vi "Do.vi"(8 "Error In":errorcluster, 10 "Actor in":refnum<class "Actor.lvclass">, 11 "CS++LNAMessage":refnum<class "CS++LNAMessage.lvclass">) -> (0 "Error Out":errorcluster, 2 "Actor out":refnum<class "Actor.lvclass">)   [LabVIEW 2016, in "CS++LNA.lvlib" / "CS++LNAMessage.lvclass"]
doc: "This VI creates the desired message object as class default object. Derives message classes need to override the <b>Parameter to Attribute.vi</b> to parse the variant attributes to the message object attribute.\n\nVI-Parameter Names of corresponding public VI of the derived actor class = Variant Attribute Names\n\nErrors (-8990, -8991, -8992) need to be handled in actor's <b>Handle Error.vi</b>\n\n(<B>Filename</B>: Actor Framework.lvlib:Message.lvclass:Do.vi)\n\nDefines what a message does when it is received by an actor. Generally, a message instructs an actor to invoke one of its methods. By default, this method does nothing. A child class must override it to define behavior. Create a child class by using the Actor Framework Message Maker dialog box."
uses:
  CS++LNAMessage.lvclass
  <vilib>/ActorFramework/Actor/Actor.lvclass
  <vilib>/ActorFramework/Message/Message.lvclass
  CS++LNAMessage.lvclass/CS++LNAMessage.ctl
  CS++LNAReturnMessage/CS++LNAReturnMessage.lvclass
  CSPP_Core/Libraries/Utilities/CS++Utilities.lvlib
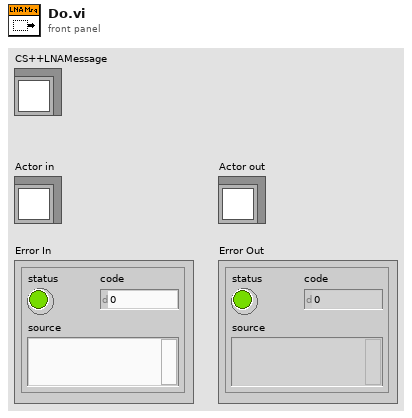
[diagram p1: front panel]
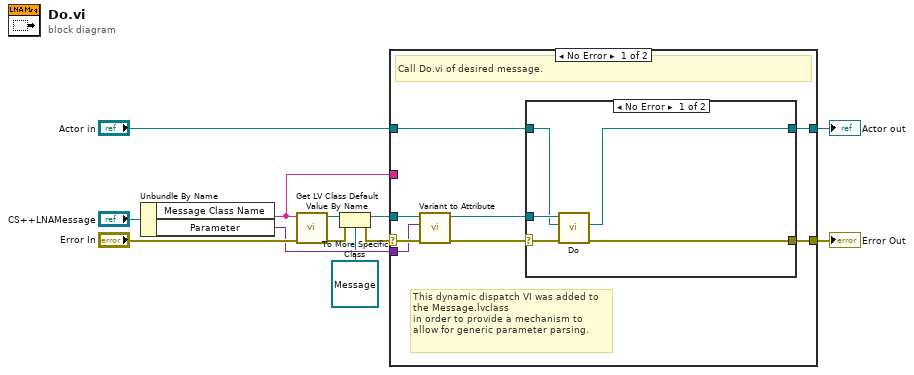
[diagram p0: block diagram]
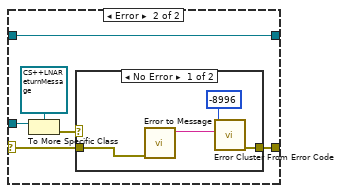
[diagram p2: hidden frame]
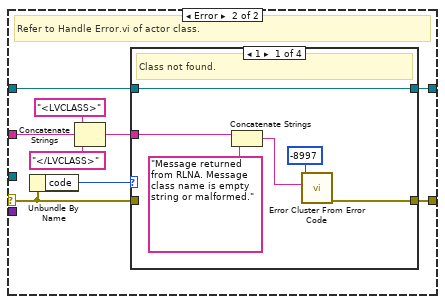
[diagram p4: hidden frame]
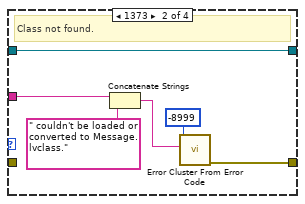
[diagram p5: hidden frame]
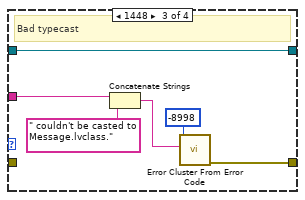
[diagram p6: hidden frame]
diagram:
  n1 = Unbundle By Name("CS++LNAMessage") -> ("Message Class Name"=w1:string, "Parameter"=w6:variant)
  n2 = call <vilib>:"Get LV Class Default Value By Name.vi"("error in (no error)"="Error In", "class name"=w1) -> ("error out"=w5:errorcluster, "object"=w9:refnum<class>)  [unwired: 8 in]
  n3 = To More Specific Class(target class=refnum<class "Message.lvclass"> refnum ("Message"), reference=w9, error in=w5) -> (specific class reference=w3:refnum<class "Message.lvclass">, error out=w2:errorcluster)
  n4 = case shown="No Error" w2 {
    selector: w2 -> [w16 w44]
    tunnel: [w20 w41] -> w12
    tunnel: "Actor in" -> [w18 w43]
    tunnel: [w19 w42] -> w10
    tunnel: w6 -> [w15 _]
    tunnel: w3 -> [w17 _]
    tunnel: w1 -> [_ w39]
    frame No Error {
      # "This dynamic dispatch VI was added to the Message.lvclass\nin order to provide a mechanism to allow for generic parameter parsing."
      # "Call Do.vi of desired message."
      n5 = call-dynamic "Variant to Attribute.vi"("Error In"=w16, "Parameter"=w15, "Message in"=w17) -> ("Error Out"=w14:errorcluster, "Message out"=w13:refnum<class "Message.lvclass">)  [unwired: 7 in]
      n6 = case shown="No Error" w14 {
        selector: w14 -> [w22 w27]
        tunnel: [w25 w28] -> w20
        tunnel: [w24 w31] -> w19
        tunnel: w13 -> [w23 w30]
        tunnel: w18 -> [w21 w31]
        frame No Error {
          n7 = call-dynamic "Do.vi"("error in (no error)"=w22, "Actor in"=w21, "Message"=w23) -> ("error out"=w25:errorcluster, "Actor out"=w24:refnum<class "Actor.lvclass">)  [unwired: 7 in]
        }
        frame Error {
          n8 = To More Specific Class(target class=refnum<class "CS++LNAReturnMessage.lvclass"> refnum ("CS++LNA.lvlib:CS++LNAReturnMessage.lvclass"), reference=w30) -> (error out=w26:errorcluster)  [unwired: 1 in, 1 out]
          n9 = case shown="No Error" w26 {
            tunnel: [w35 w36] -> w28
            tunnel: w27 -> [w33 w36]
            frame No Error {
              n10 = call "Error to Message.vi"("Error In"=w33) -> ("Error Message"=w32:string)  [unwired: 9 in, 1 out]
              n11 = call <vilib>:"Error Cluster From Error Code.vi"("error message (\"\")"=w32, "error code (0)"=-8996) -> ("error out"=w35:errorcluster)  [unwired: 7 in]
            }
            frame Error {
            }
          }
        }
      }
    }
    frame Error {
      # "Refer to Handle Error.vi of actor class."
      n12 = Unbundle By Name(w44) -> ("code"=w45:i32)
      n13 = Concatenate Strings("<LVCLASS>" ("string"), w39, "</LVCLASS>" ("string")) -> (w37:string)
      n14 = case shown="1" w45 {
        tunnel: [w51 w57 w63 w65] -> w42
        tunnel: w43 -> [w51 w57 w63 w65]
        tunnel: [w48 w54 w59 w64] -> w41
        tunnel: w44 -> [_ _ _ w64]
        tunnel: w37 -> [w46 w52 w62 _]
        frame 1 {
          # "Class not found."
          n15 = Concatenate Strings(w46, "Message returned from RLNA. Message class name is empty string or malformed.") -> (w49:string)
          n16 = call <vilib>:"Error Cluster From Error Code.vi"("error message (\"\")"=w49, "error code (0)"=-8997) -> ("error out"=w48:errorcluster)  [unwired: 7 in]
        }
        frame 1373 {
          # "Class not found."
          n17 = Concatenate Strings(w52, " couldn't be loaded or converted to Message.lvclass.") -> (w55:string)
          n18 = call <vilib>:"Error Cluster From Error Code.vi"("error message (\"\")"=w55, "error code (0)"=-8999) -> ("error out"=w54:errorcluster)  [unwired: 7 in]
        }
        frame 1448 {
          # "Bad typecast"
          n19 = Concatenate Strings(w62, " couldn't be casted to Message.lvclass.") -> (w60:string)
          n20 = call <vilib>:"Error Cluster From Error Code.vi"("error message (\"\")"=w60, "error code (0)"=-8998) -> ("error out"=w59:errorcluster)  [unwired: 7 in]
        }
        frame Default {
          # "unkonw error"
        }
      }
    }
  }
  "Error Out" <- w12
  "Actor out" <- w10
